vi "Receive Response.vi"(8 "error in (no error)":errorcluster, 10 "Command in":T1, 11 "Hitronics in":refnum<class "Hitronics.lvclass">) -> (0 "error out":errorcluster, 2 "Response":string, 3 "Hitronics out":refnum<class "Hitronics.lvclass">)   [LabVIEW 2018, in "Hitronics.lvlib" / "Hitronics.lvclass"]
doc: "Read response data from laser"
uses:
  Hitronics.lvclass
  PPLs/Laser/Parent/Laser.lvlibp/Custom Controls/Command List.ctl
  PPLs/Laser/Parent/Laser.lvlibp/Laser.lvclass
  C:/AME Test Engineering/LabVIEW/PPLs/Laser/Parent/Laser.lvlibp/Laser.lvclass
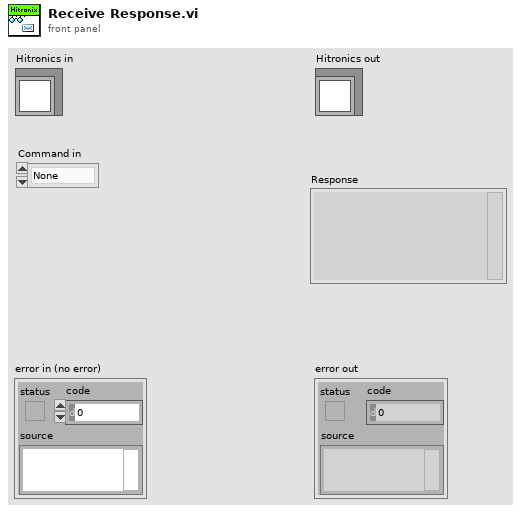
[diagram p1: front panel]
types:
  T1 = typedef "Laser.lvlibp/Laser.lvclass/Command List.ctl" = enum16{"None", "Config?", "Volt?", "ThCase?", "STS?", "Mon?", "Help?", "HB", "Verbose", "Spnt", "Ext", "PRF", "Start", "Stop", "PRF?", "State?", "Status?", "Stat?", "Read HB", "Logon", "Poutmax", "saveconfig", "Reset", "Poutmax?", "PoutCommandMax", "PoutCommandMax?", "FreqMin", "FreqMin?"}
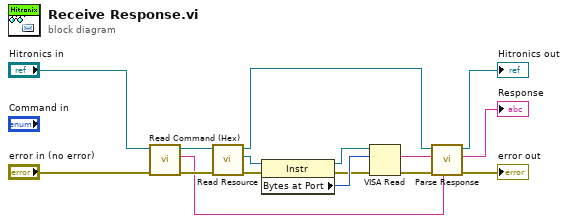
[diagram p0: block diagram]
diagram:
  n1 = call-dynamic "Read Command (Hex).vi"("error in (no error)"="error in (no error)", "Hitronics in"="Hitronics in") -> ("error out"=w9:errorcluster, "Command (Hex)"=w7:string, "Hitronics out"=w8:refnum<class "Hitronics.lvclass">)  [unwired: 7 in]
  n2 = call "Read Resource.vi"("error in (no error)"=w9, "Laser in"=w8) -> ("error out"=w12:errorcluster, "Resource"=w13:refnum<visa-resource-name>, "Laser out"=w6:refnum<class "Hitronics.lvclass">)  [unwired: 7 in]
  n3 = property class="Instr"(reference=w13, error in=w12) -> (reference out=w15:refnum<visa-resource-name>, error out=w14:errorcluster, "Bytes at Port"=w16:u32)
  n4 = VISA Read(VISA resource name=w15, byte count=w16, error in (no error)=w14) -> (read buffer=w5:string, error out=w3:errorcluster)  [unwired: 2 out]
  n5 = call "Parse Response.vi"("Command String (Hex)"=w7, "error in (no error)"=w3, "Response String (Hex)"=w5, "Hitronics in"=w6) -> ("error out"=→"error out":errorcluster, "Response"=→"Response":string, "Hitronics out"=→"Hitronics out":refnum<class "Hitronics.lvclass">)  [unwired: 5 in]
